vi "checkPortMissing.vi"(8 "Required":bool[](array[boolean]), 11 "NXT/EV3":T1) -> (0 "Success":bool, 3 "NXT/EV3":T1)   [LabVIEW 2013]
uses:
  <vilib>/NXT/Subs/LVHSConnector.ctl
  <vilib>/NXT/LegoClasses/BrickReference/BrickReference.lvclass
  <vilib>/NXT/Dual Mode Library/Advanced/NXTFlag_Get_Integer.vi
  <vilib>/NXT/Dual Mode Library/Display/drawPicture.vi
  <vilib>/NXT/Dual Mode Library/Display/drawText_Center.vi
  <vilib>/NXT/Dual Mode Library/Waits/Wait_Num.vi
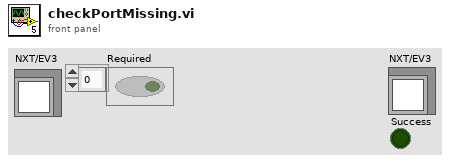
[diagram p1: front panel]
types:
  T1 = typedef "LVHSConnector.ctl" = refnum<class "BrickReference.lvclass">
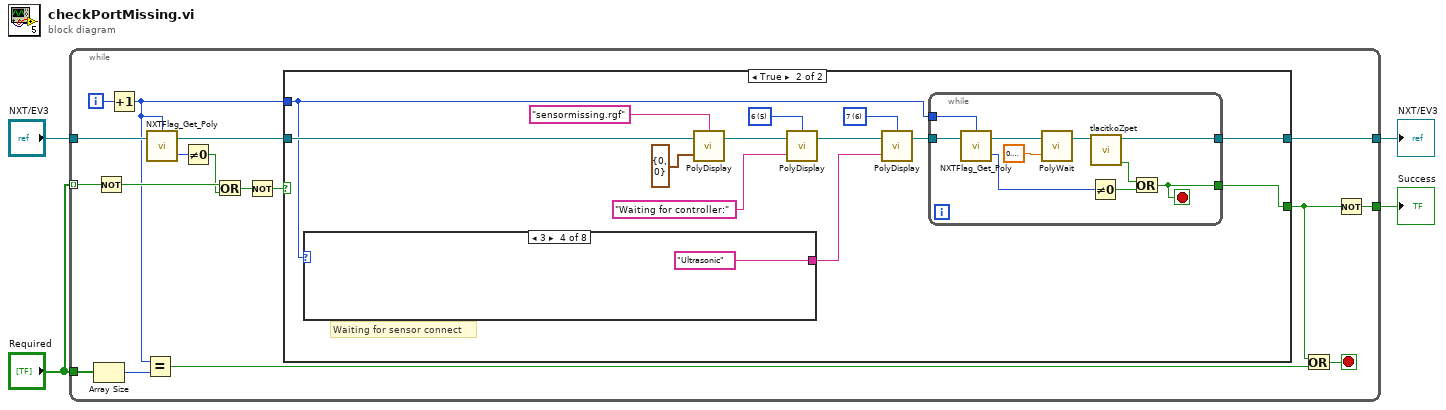
[diagram p0: block diagram]
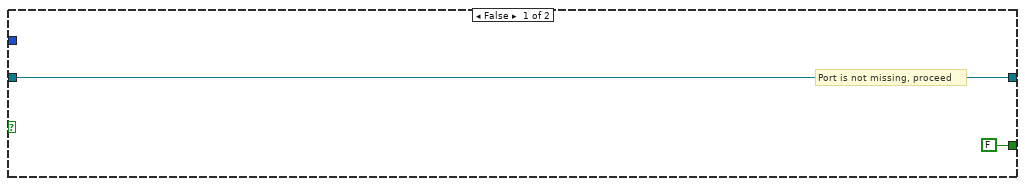
[diagram p2: hidden frame]
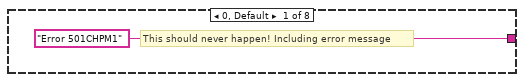
[diagram p3: hidden frame]
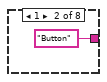
[diagram p4: hidden frame]
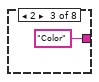
[diagram p5: hidden frame]
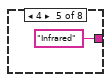
[diagram p6: hidden frame]
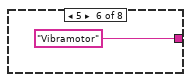
[diagram p7: hidden frame]
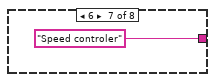
[diagram p8: hidden frame]
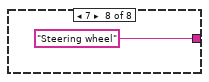
[diagram p9: hidden frame]
diagram:
  n1 = while {
    tunnel: [w12] -> w3
    tunnel: "NXT/EV3" -> [w21]
    tunnel: "Required" -> [w18] mode=indexing
    tunnel: "Required" -> [w8]
    tunnel: [w5] -> w1
    i -> [w20]
    stop <- w7 stop-if-true
    n2 = Array Size(array=w8) -> (size(s)=w9:i32)
    n3 = Not(x=w18) -> (.not. x?=w17:bool)
    n4 = Increment(x=w20) -> (x+1=w10:i32)
    n5 = Equal?(x=w10, y=w9) -> (x = y?=w11:bool)
    n6 = call-poly <vilib>:"NXTFlag_Get_Poly.vi"("NXT/EV3"=w21, "NXT/EV3 Flag Number"=w10) -> ("Flag Value"=w19:i32, "NXT/EV3"=w13:T1)  [unwired: 1 in]
    n7 = Not Equal To 0?(x=w19) -> (x != 0?=w16:bool)
    n8 = Or(x=w17, y=w16) -> (x .or. y?=w15:bool)
    n9 = Not(x=w15) -> (.not. x?=w14:bool)
    n10 = case shown="True" w14 {
      tunnel: w13 -> [w23 w34]
      tunnel: [w23 w27] -> w12
      tunnel: w10 -> [_ w25]
      tunnel: [FALSE w24] -> w6
      frame False {
        # "Port is not missing, proceed"
      }
      frame True {
        w28 = i16 6 items=["1", "2", "3", "4", "5", "6", "7", "8", "9", "10", "11", "12"] ("Line")
        w32 = i16 5 items=["1", "2", "3", "4", "5", "6", "7", "8", "9", "10", "11", "12"] ("Line")
        # "Waiting for sensor connect"
        n11 = case shown="3" w25 {
          tunnel: ["Error 501CHPM1" ("Text") "Button" ("Text") "Color" ("Text") "Ultrasonic" ("Text") "Infrared" ("Text") "Vibramotor" ("Text") "Speed controler" ("Text") "Steering wheel" ("Text")] -> w26
          frame 0, Default {
            # "This should never happen! Including error message"
          }
          frame 1 {
          }
          frame 2 {
          }
          frame 3 {
          }
          frame 4 {
          }
          frame 5 {
          }
          frame 6 {
          }
          frame 7 {
          }
        }
        n12 = call-poly <vilib>:"PolyDisplay.vi"("Origin"=cluster{"X":i16, "Y":i16} {"X"=0, "Y"=0}, "NXT/EV3"=w34, "Filename (*.ric/*.rgf)"="sensormissing.rgf") -> ("NXT/EV3"=w33:T1)  [unwired: 1 in]
        n13 = call-poly <vilib>:"PolyDisplay.vi"("Text"="Waiting for controller:", "NXT/EV3"=w33, "Line"=w32) -> ("NXT/EV3"=w30:T1)  [unwired: 1 in]
        n14 = call-poly <vilib>:"PolyDisplay.vi"("Text"=w26, "NXT/EV3"=w30, "Line"=w28) -> ("NXT/EV3"=w29:T1)  [unwired: 1 in]
        n15 = while {
          tunnel: w29 -> [w46]
          tunnel: [w40] -> w27
          tunnel: w25 -> [w44]
          tunnel: [w37] -> w24
          stop <- w37 stop-if-true
          n16 = call-poly <vilib>:"NXTFlag_Get_Poly.vi"("NXT/EV3"=w46, "NXT/EV3 Flag Number"=w44) -> ("Flag Value"=w43:i32, "NXT/EV3"=w45:T1)  [unwired: 1 in]
          n17 = call-poly <vilib>:"PolyWait.vi"("Time (1 sec)"=sgl 0.1, "NXT/EV3"=w45) -> ("NXT/EV3"=w41:T1)  [unwired: 2 in]
          n18 = Not Equal To 0?(x=w43) -> (x != 0?=w38:bool)
          n19 = call "tlacitkoZpet.vi"("NXT/EV3"=w41) -> ("Boolean"=w39:bool, "NXT/EV3 2"=w40:T1)  [unwired: 9 in]
          n20 = Or(x=w39, y=w38) -> (x .or. y?=w37:bool)
        }
      }
    }
    n21 = Or(x=w6, y=w11) -> (x .or. y?=w7:bool)
    n22 = Not(x=w6) -> (.not. x?=w5:bool)
  }
  "NXT/EV3" <- w3
  "Success" <- w1
